vi "Standalone Device FP.vi"() -> ()   [LabVIEW 2015]
panel:
  out "RPM":dbl(knob) scale=0.0..10.0
  in  "Ranges":u16(ring) items=["5V", "10V"]
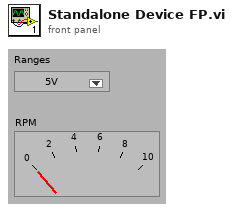
[diagram p1: front panel]
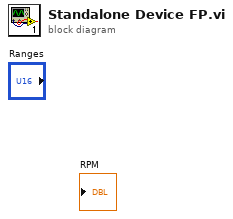
[diagram p0: block diagram]
diagram:
